vi "Pipe Var Intf - Test Wait For Connect.vi"() -> ()   [LabVIEW 2020, in "GOLPI library.lvlib"]
uses:
  GOLPI library.lvlib
panel:
  out "read bytes":u32
  in  "bytes to read (0)":i32
  out "written bytes":u32
  out "write cycle":i32
  in  "btn read":bool
  in  "write block size":i32
  out "handle":i32
  in  "btn stop client":bool
  in  "btn close":bool
  out "error out 2":errorcluster
  in  "btn open":bool
  in  "stop":bool
  in  "pipe name in (leave empty to generate random name)":string="\\\\.\\Pipe\\GOLPI_Variable_Pipe"
  out "error out":errorcluster
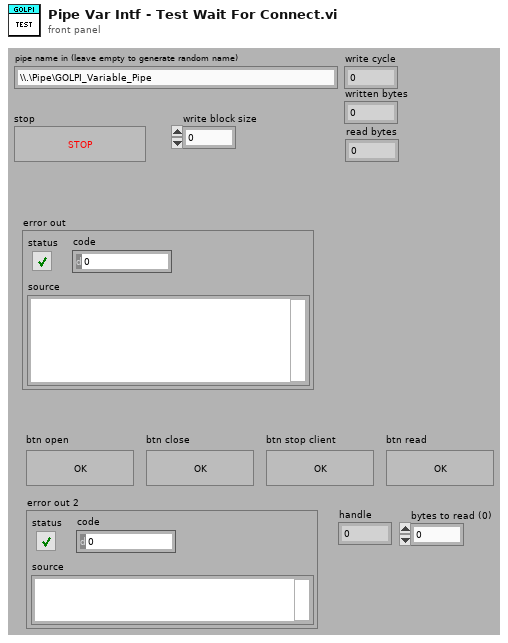
[diagram p1: front panel]
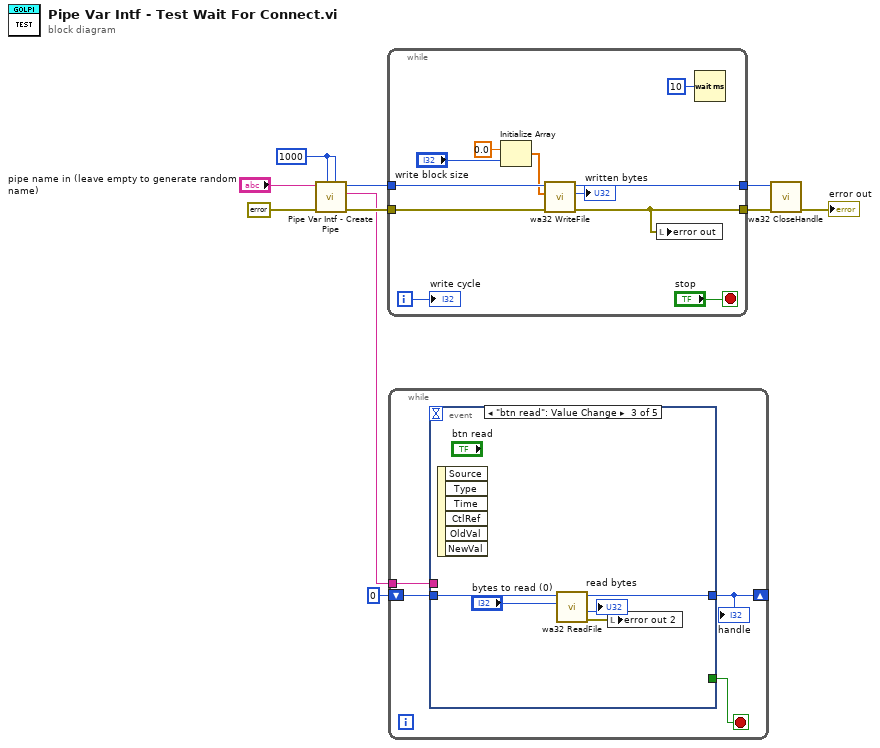
[diagram p0: block diagram]
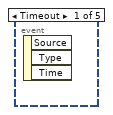
[diagram p2: hidden frame]
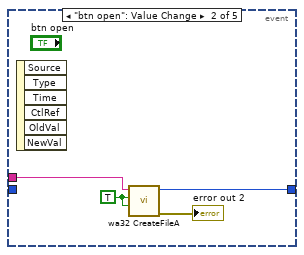
[diagram p3: hidden frame]
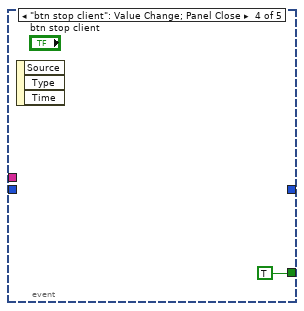
[diagram p4: hidden frame]
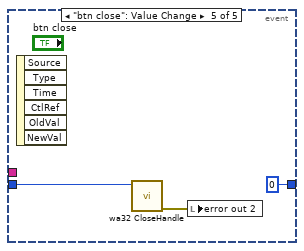
[diagram p5: hidden frame]
diagram:
  w1 = u32 1000 ("inBufferSize (256k)")
  n1 = call "Pipe Var Intf - Create Pipe.vi"("outBufferSize (256k)"=w1, "inBufferSize (256k)"=w1, "error in (no error)"=errorcluster {"status"=FALSE, "code"=0, "source"=""} ("error out"), "pipe name in (leave empty to generate random name)"="pipe name in (leave empty to generate random name)") -> ("error out"=w7:errorcluster, "pipe name out"=w2:string, "pipe handle out"=w5:i32)  [unwired: 5 in]
  n2 = while {
    tunnel: w5 -> [w19]
    tunnel: [w13] -> w4
    tunnel: w7 -> [w20]
    tunnel: [w11] -> w6
    i -> [w14]
    stop <- "stop" stop-if-true
    n3 = Initialize Array(0.0 ("element"), "write block size") -> (w17:dbl[])
    n4 = call "wa32 WriteFile.vi"("error in"=w20, "data (empty)"=w17, "handle"=w19) -> ("error out"=w11:errorcluster, "written bytes"=→"written bytes":u32, "handle out"=w13:i32)  [unwired: 6 in]
    n5 = local write "error out"(w11) -> ()
    n6 = Wait (ms)(milliseconds to wait=u32 10) -> ()  [unwired: 1 out]
    "write cycle" <- w14
  }
  n7 = while {
    shift-right: [w25] -> _
    shift-left: 0 ("handle") -> [w24]
    tunnel: w2 -> [w23]
    stop <- w22 stop-if-true
    n8 = event shown="[2] \"btn read\": Value Change" {
      selector: _ -> [_ _ _ _ _]
      dyn-events: _ -> [_ _ _ _ _]
      timeout: _ -> [_ _ _ _ _]
      tunnel: [_ w28 w33 _ 0 ("handle")] -> w25
      tunnel: w24 -> [_ _ w34 _ w38]
      tunnel: w23 -> [_ w27 _ _ _]
      tunnel: [_ _ _ TRUE _] -> w22
      event Timeout {
        n9 = event-data() -> ()  [unwired: 1 in, 3 out]
      }
      event "btn open": Value Change {
        w26 = TRUE ("read")
        n10 = event-data() -> ()  [unwired: 1 in, 6 out]
        n11 = call "wa32 CreateFileA.vi"("write"=w26, "read"=w26, "file path"=w27) -> ("error out"=→"error out 2":errorcluster, "handle"=w28:i32)  [unwired: 7 in]
      }
      event "btn read": Value Change {
        n12 = event-data() -> ()  [unwired: 1 in, 6 out]
        n13 = call "wa32 ReadFile.vi"("bytes to read (0)"="bytes to read (0)", "handle"=w34) -> ("error out"=w32:errorcluster, "read bytes"=→"read bytes":u32, "handle out"=w33:i32)  [unwired: 5 in, 2 out]
        n14 = local write "error out 2"(w32) -> ()
      }
      event "btn stop client": Value Change; Panel Close {
        n15 = event-data() -> ()  [unwired: 1 in, 3 out]
      }
      event "btn close": Value Change {
        n16 = event-data() -> ()  [unwired: 1 in, 6 out]
        n17 = call "wa32 CloseHandle.vi"("handle"=w38) -> ("error out"=w36:errorcluster)  [unwired: 10 in]
        n18 = local write "error out 2"(w36) -> ()
      }
    }
    "handle" <- w25
  }
  n19 = call "wa32 CloseHandle.vi"("error in"=w6, "handle"=w4) -> ("error out"=→"error out":errorcluster)  [unwired: 9 in]
